vi "List Managers.vi"(11 "SMOConfigManager in":refnum<class "SMOConfigManager.lvclass">) -> (2 "List":refnum<class "SMOConfigManager.lvclass">[](array[class]), 3 "SMOConfigManager out":refnum<class "SMOConfigManager.lvclass">)   [LabVIEW 2013, in "SMOConfigManager.lvclass"]
uses:
  SMOConfigManager.lvclass
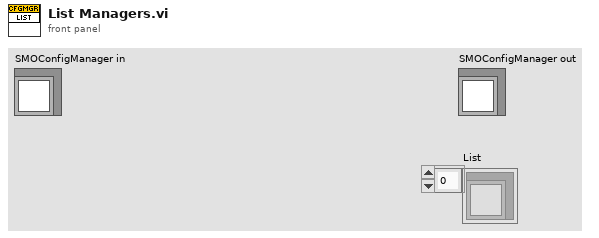
[diagram p1: front panel]
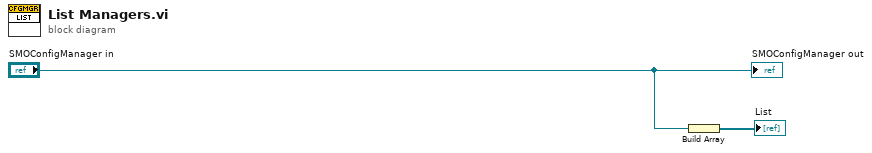
[diagram p0: block diagram]
diagram:
  n1 = Build Array("SMOConfigManager in") -> (→"List":refnum<class "SMOConfigManager.lvclass">[])
  "SMOConfigManager out" <- "SMOConfigManager in"
